vi "06_jednoduche_simulovani_ujizdejiciho_signalu.vi"() -> ()   [LabVIEW 2019]
uses:
  <vilib>/measure/NI_MABase.lvlib
panel:
  out "Waveform Graph":dbl[](graph)
  in  "stop":bool
  out "dt (s)":dbl=0.001
  out "Vzorkovaci Frekvence (N)":dbl=1000.0
  in  "Amplituda sumu":dbl=0.9999999999999999 format="%.2p"
  in  "Info o vzorkovani":T1={"Vzorkovaci frekvence"=1000.0, "Pocet vzorku v okne"=1000.0} {"Vzorkovaci frekvence" format="%.2p"}
  in  "Amplituda":dbl=10.0 format="%0.2p"
  in  "Frekvence":dbl=10.0 format="%0.2p"
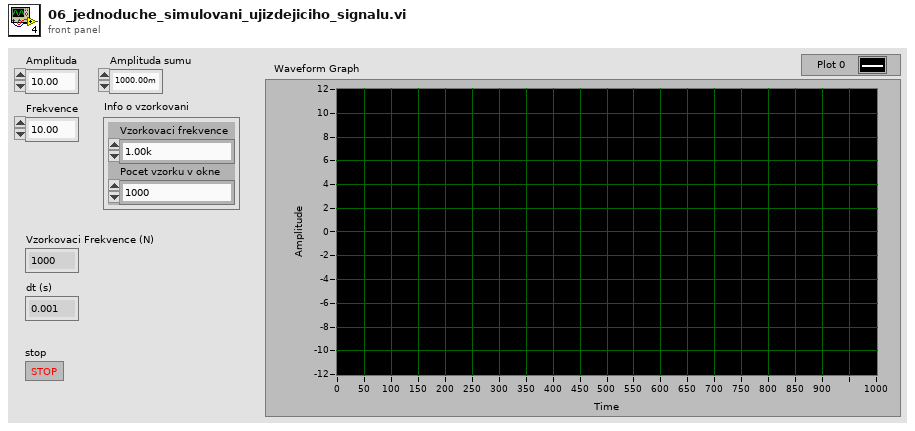
[diagram p1: front panel]
types:
  T1 = cluster{"Vzorkovaci frekvence":dbl, "Pocet vzorku v okne":dbl}
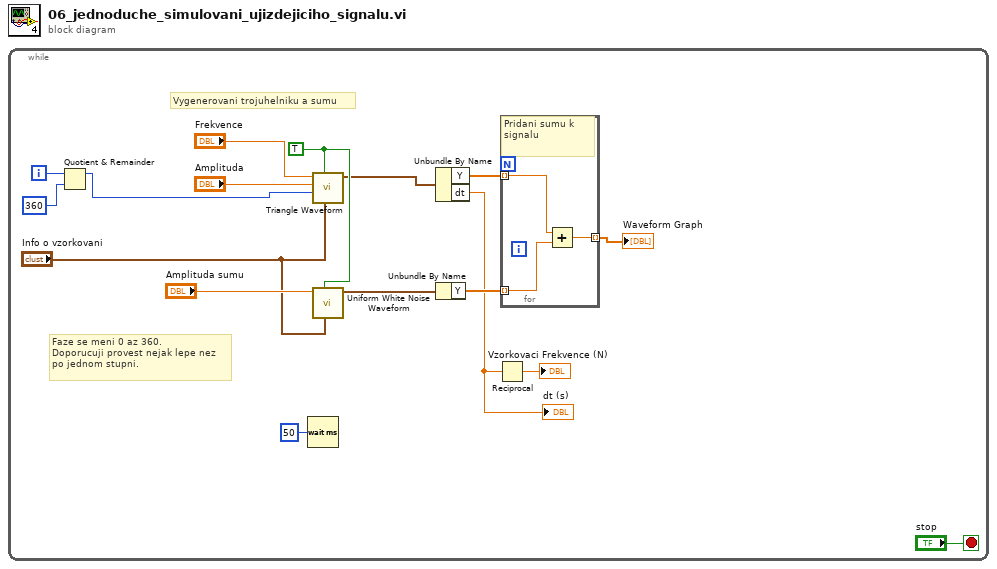
[diagram p0: block diagram]
diagram:
  n1 = while {
    i -> [w4]
    stop <- "stop" stop-if-true
    w14 = TRUE ("reset signal")
    # "Faze se meni 0 az 360.\nDoporucuji provest nejak lepe nez\npo jednom stupni."
    # "Vygenerovani trojuhelniku a sumu"
    n2 = Quotient & Remainder(x=w4, y=360) -> (x-y*floor(x/y)=w2:i32)  [unwired: 1 out]
    n3 = Wait (ms)(milliseconds to wait=u32 50) -> ()  [unwired: 1 out]
    n4 = call <vilib>:"Triangle Waveform.vi"("sampling info"="Info o vzorkovani", "reset signal"=w14, "phase"=w2, "amplitude"="Amplituda", "frequency"="Frekvence") -> ("signal out"=w10:waveform(dbl))  [unwired: 5 in, 1 out]
    n5 = call <vilib>:"Uniform White Noise Waveform.vi"("sampling info"="Info o vzorkovani", "reset signal"=w14, "amplitude"="Amplituda sumu") -> ("signal out"=w13:waveform(dbl))  [unwired: 7 in, 1 out]
    n6 = Unbundle By Name(w10) -> ("Y"=w12:dbl[], "dt"=w9:dbl)
    "dt (s)" <- w9
    n7 = Unbundle By Name(w13) -> ("Y"=w11:dbl[])
    n8 = Reciprocal(x=w9) -> (1/x=→"Vzorkovaci Frekvence (N)":dbl)
    n9 = for {
      tunnel: w12 -> [w19] mode=indexing
      tunnel: w11 -> [w20] mode=indexing
      tunnel: [w18] -> w5 mode=indexing
      # "Pridani sumu k signalu"
      n10 = Add(x=w19, y=w20) -> (x+y=w18:dbl)
    }
    "Waveform Graph" <- w5
  }
